vi "BypassControl.vi"(6 "Cutoff":dbl=0.15 format="%#_13g", 8 "Skip":dbl, 10 "DesiredInput":dbl, 11 "CurrentInput":dbl) -> (3 "SetMotor":dbl)   [LabVIEW 2013]
doc: "Skips motor values that are, for all intents and purposes, 0. This VI includes trapezoidal acceleration."
panel:
  in  "LoopTime":dbl
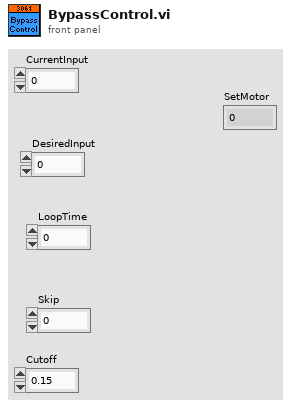
[diagram p1: front panel]
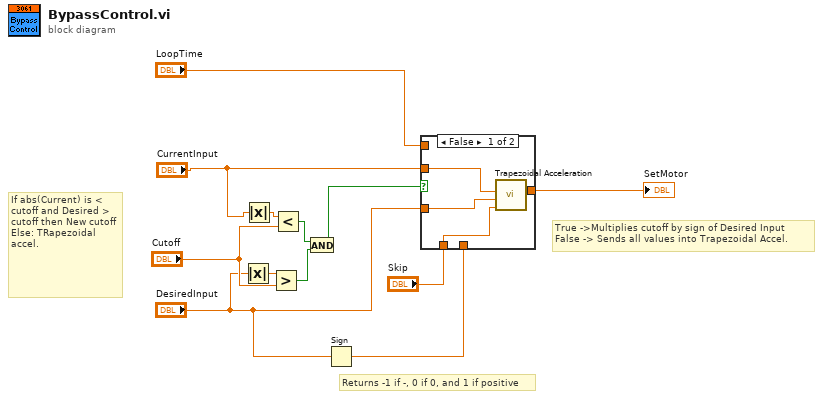
[diagram p0: block diagram]
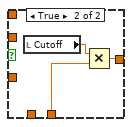
[diagram p2: hidden frame]
diagram:
  # "If abs(Current) is < cutoff and Desired > cutoff then New cutoff\nElse: TRapezoidal accel."
  # "True ->Multiplies cutoff by sign of Desired Input \nFalse -> Sends all values into Trapezoidal Accel."
  # "Returns -1 if -, 0 if 0, and 1 if positive"
  n1 = Absolute Value(x="DesiredInput") -> (abs(x)=w10:dbl)
  n2 = Absolute Value(x="CurrentInput") -> (abs(x)=w11:dbl)
  n3 = Greater?(x=w10, y="Cutoff") -> (0:w8:bool)
  n4 = Less?(x=w11, y="Cutoff") -> (x < y?=w9:bool)
  n5 = And(x=w9, y=w8) -> (x .and. y?=w7:bool)
  n6 = Sign(1:"DesiredInput") -> (0:w5:dbl)
  n7 = case shown="False" w7 {
    tunnel: "DesiredInput" -> [w15 _]
    tunnel: "CurrentInput" -> [w16 _]
    tunnel: [w14 w19] -> w4
    tunnel: w5 -> [_ w18]
    tunnel: "LoopTime" -> [_ _]
    tunnel: "Skip" -> [w13 _]
    frame False {
      n8 = call "Trapezoidal Acceleration.vi"("Skip"=w13, "Desired"=w15, "Actual"=w16) -> ("New Actual"=w14:dbl)  [unwired: 8 in]
    }
    frame True {
      n9 = local read "Cutoff"() -> (w17:dbl)
      n10 = Multiply(x=w17, y=w18) -> (x*y=w19:dbl)
    }
  }
  "SetMotor" <- w4
